vi "Function_Yellow Spot.vi"(0 "Image Src In":T4, 5 "Data Cluster In":cluster{"Name":string, "Variant In":variant}, 7 "CoordSys In":T1 {"Measurement System"."Axis Reference" items=["Direct", "Indirect"]; "Measurement System"."Angle (deg)" format="%.2f"; "Measurement System"."Origin"."Y" format="%.2f"; "Measurement System"."Origin"."X" format="%.2f"; "Reference System"."Axis Reference" items=["Direct", "Indirect"]; "Reference System"."Angle (deg)" format="%.2f"; "Reference System"."Origin"."Y" format="%.2f"; "Reference System"."Origin"."X" format="%.2f"}, 9 "Center(Annulus)":cluster{"X":sgl, "Y":sgl} {"Y" format="%.2f"; "X" format="%.2f"}, 11 "Error in":errorcluster) -> (4 "Objects":T3(array[cluster]) {"Area" format="%.2f"; "Object Center"."Y" format="%.2f"; "Object Center"."X" format="%.2f"}, 6 "Result(Yellow)":cluster{"Name":string, "NG?":bool, "Score":dbl}, 10 "ROI Out":T2 {"Contours"."Type" items=["No Selection", "Point", "Line", "Rectangle", "Oval", "Polygon", "Free", "Annulus", "Unused2", "Unused3", "Broken Line", "Free Hand Line", "Rotated Rectangle"]}, 14 "Time":u32, 15 "Error out":errorcluster)   [LabVIEW 2013]
uses:
  <vilib>/vision/Image Controls.llb/IMAQ Image.ctl
  Control/Control_Yellow Spot.ctl
  <vilib>/vision/NI_Vision_Development_Module.lvlib
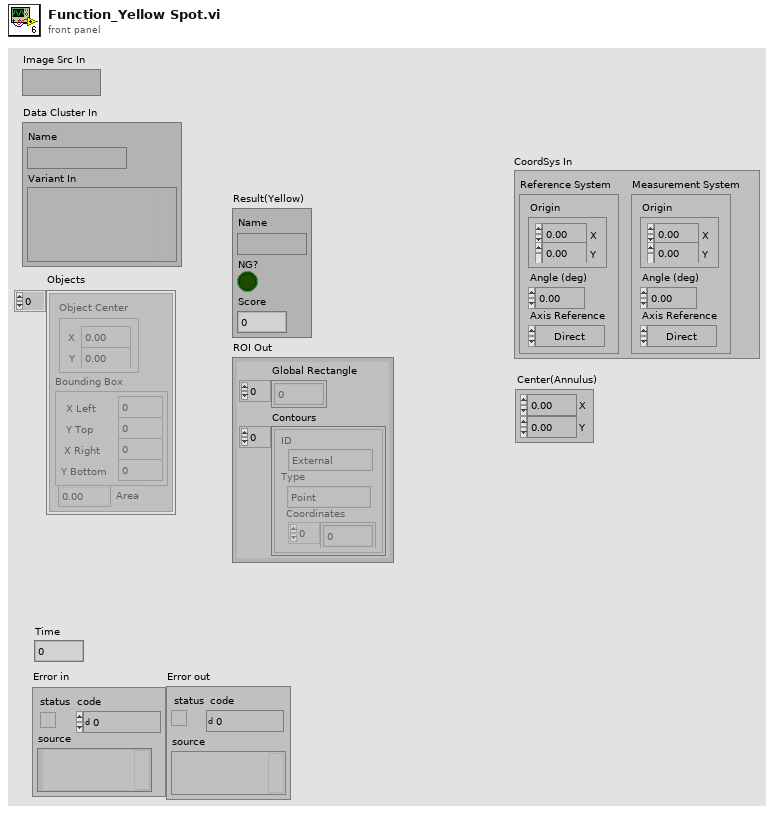
[diagram p1: front panel]
types:
  T1 = typedef "IMAQ Coordinate System" = cluster{"Reference System":cluster{"Origin":cluster{"X":sgl, "Y":sgl}, "Angle (deg)":sgl, "Axis Reference":u32}, "Measurement System":cluster{"Origin":cluster{"X":sgl, "Y":sgl}, "Angle (deg)":sgl, "Axis Reference":u32}}
  T2 = cluster{"Global Rectangle":i32[], "Contours":cluster{"ID":enum32{"External", "Internal"}, "Type":u32, "Coordinates":i32[]}[]}
  T3 = cluster{"Object Center":cluster{"X":dbl, "Y":dbl}, "Bounding Box":cluster{"X Left":dbl, "Y Top":dbl, "X Right":dbl, "Y Bottom":dbl}, "Area":dbl}[]
  T4 = typedef "IMAQ Image.ctl" = refnum<image>
  T5 = typedef "Control_Yellow Spot.ctl" = cluster{"Name":string, "ROI":cluster{"Global Rectangle":i32[], "Contours":cluster{"ID":enum32{"External", "Internal"}, "Type":u32, "Coordinates":i32[]}[]}, "Magnification(独闯)":i32, "»Ö­È(¶À´³)":i16, "Settings(独闯)":cluster{"Objects":enum16{"Bright Objects", "Dark Objects"}, "Threshold":i32, "Min Object Size":bool, "Min Size":i32, "Max Object Size":bool, "Max Size":i32}}
  T6 = cluster{"Objects":enum16{"Bright Objects", "Dark Objects"}, "Threshold":i32, "Min Object Size":bool, "Min Size":i32, "Max Object Size":bool, "Max Size":i32}
  T7 = cluster{"ID":enum32{"External", "Internal"}, "Type":u32, "Coordinates":i32[]}[]
  T8 = cluster{"ID":enum32{"External", "Internal"}, "Type":u32, "Coordinates":i32[]}
  T9 = cluster{"Origin":cluster{"X":sgl, "Y":sgl}, "Angle (deg)":sgl, "Axis Reference":u32}
  T10 = typedef "ROI Descriptor" = cluster{"Global Rectangle":i32[], "Contours":cluster{"ID":enum32{"External", "Internal"}, "Type":u32, "Coordinates":i32[]}[]}
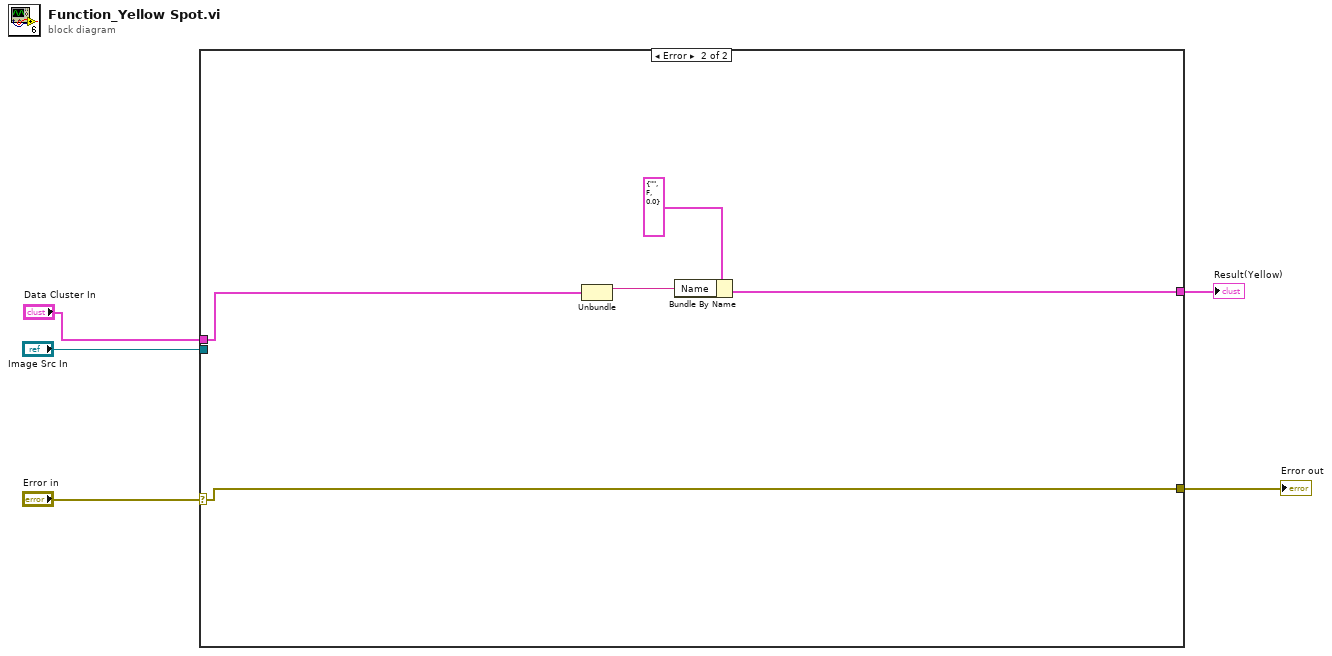
[diagram p0: block diagram]
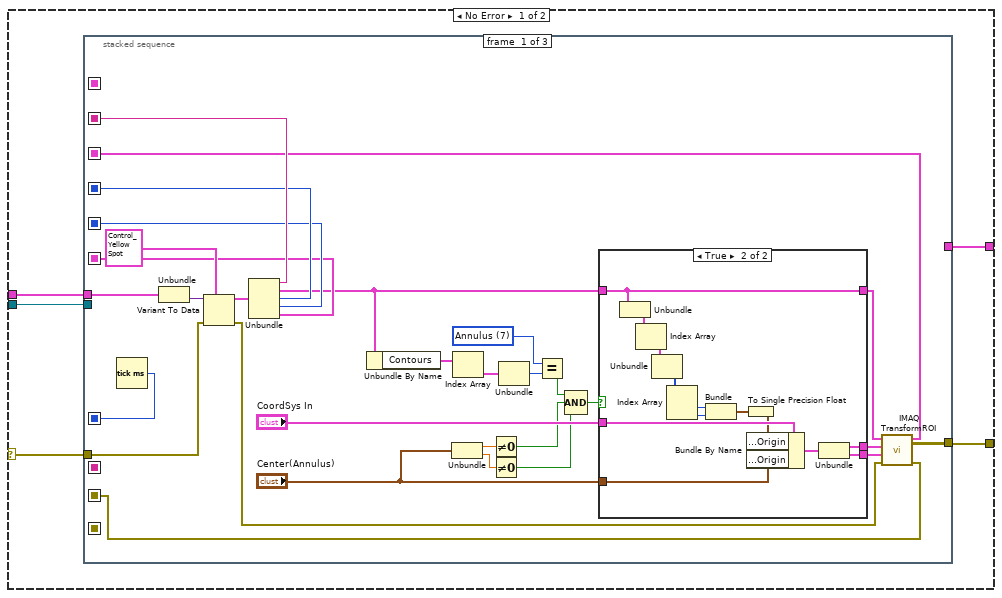
[diagram p2: hidden frame]
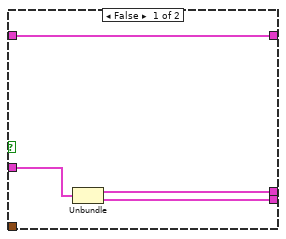
[diagram p3: hidden frame]
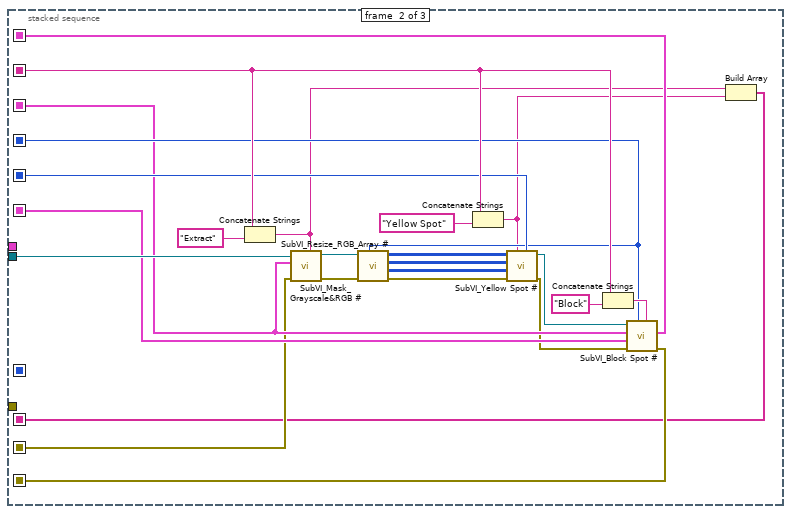
[diagram p4: hidden frame]
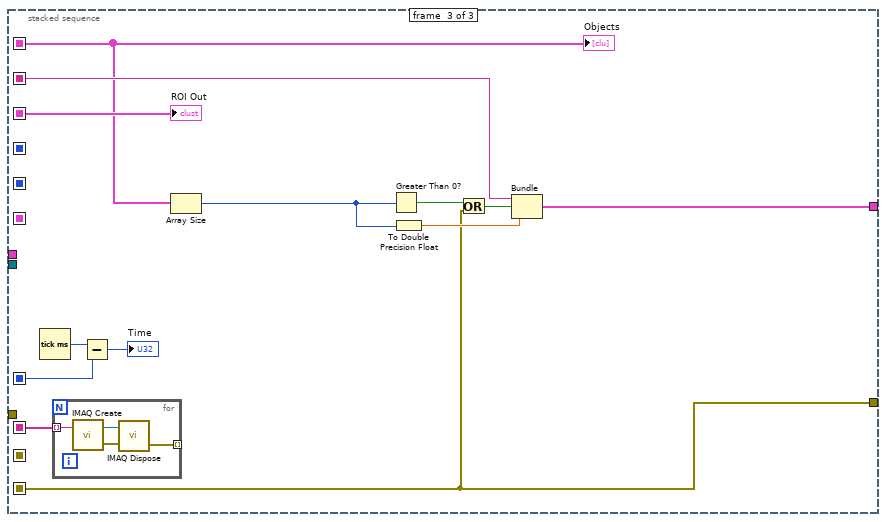
[diagram p5: hidden frame]
diagram:
  n1 = case shown="Error" "Error in" {
    selector: "Error in" -> [w8 w102]
    tunnel: [w10 w102] -> w5
    tunnel: "Image Src In" -> [w9 _]
    tunnel: [w7 w98] -> w2
    tunnel: "Data Cluster In" -> [w6 w99]
    frame No Error {
      n2 = stacked-sequence {
        seq-local: [w36 _ _] -> [_ w68 w90]
        seq-local: [w23 _ _] -> [_ w64 w91]
        seq-local: [w35 _ _] -> [_ w66 _]
        seq-local: [w34 _ _] -> [_ w67 _]
        seq-local: [w33 _ _] -> [_ w65 _]
        seq-local: [_ w62 _] -> [_ _ w86]
        seq-local: [_ w61 _] -> [_ _ w89]
        seq-local: [w32 _ _] -> [_ _ w84]
        seq-local: [w12 _ _] -> [_ w60 _]
        seq-local: [_ w57 _] -> [_ _ w82]
        tunnel: w8 -> [w14 _ _]
        tunnel: [_ _ w86] -> w10
        tunnel: w9 -> [_ w73 _]
        tunnel: [_ _ w81] -> w7
        tunnel: w6 -> [w11 _ _]
        frame #0 {
          w28 = u32 7 items=["No Selection", "Point", "Line", "Rectangle", "Oval", "Polygon", "Freehand Region", "Annulus", "Unused2", "Unused3", "Broken Line", "Freehand Line", "Rotated Rectangle"] ("Type")
          n3 = Tick Count (ms)() -> (millisecond timer value=w32:u32)
          n4 = Unbundle(w11) -> ("Variant In"=w38:variant)  [unwired: 1 out]
          n5 = Variant To Data(error in=w14, type=T5 {"Name"="", "ROI"={"Global Rectangle"=[], "Contours"=[]}, "Magnification(独闯)"=0, "»Ö­È(¶À´³)"=40, "Settings(独闯)"={"Objects"=enum."Bright Objects", "Threshold"=128, "Min Object Size"=FALSE, "Min Size"=3, "Max Object Size"=FALSE, "Max Size"=100}} ("独闯_Setting"), Variant=w38) -> (data=w37:T5, error out=w13:errorcluster)
          n6 = Unbundle(w37) -> ("Name"=w36:string, "ROI"=w24:T2, "Magnification(独闯)"=w35:i32, "»Ö­È(¶À´³)"=w34:i16, "Settings(独闯)"=w33:T6)
          n7 = Unbundle By Name(w24) -> ("Contours"=w26:T7)
          n8 = Unbundle("Center(Annulus)") -> ("X"=w20:sgl, "Y"=w19:sgl)
          n9 = Index Array(array=w26) -> (element=w27:T8)  [unwired: 1 in]
          n10 = Not Equal To 0?(x=w20) -> (x != 0?=w17:bool)
          n11 = Not Equal To 0?(x=w19) -> (x != 0?=w16:bool)
          n12 = Unbundle(w27) -> ("Type"=w29:u32)  [unwired: 2 out]
          n13 = Equal?(x=w28, y=w29) -> (x = y?=w18:bool)
          n14 = Compound Arithmetic op=AND(w18, w17, w16) -> (w15:bool)
          n15 = case shown="True" w15 {
            tunnel: "CoordSys In" -> [w43 w56]
            tunnel: [w42 w50] -> w30
            tunnel: [w41 w49] -> w31
            tunnel: "Center(Annulus)" -> [_ w53]
            tunnel: w24 -> [w40 w44]
            tunnel: [w40 w44] -> w22
            frame False {
              n16 = Unbundle(w43) -> ("Reference System"=w42:T9, "Measurement System"=w41:T9)
            }
            frame True {
              n17 = Unbundle(w44) -> ("Contours"=w48:T7)  [unwired: 1 out]
              n18 = Index Array(array=w48) -> (element=w47:T8)  [unwired: 1 in]
              n19 = Unbundle(w47) -> ("Coordinates"=w46:i32[])  [unwired: 2 out]
              n20 = Index Array(array=w46) -> (element #1=w55:i32, element #2=w54:i32)  [unwired: 2 in]
              n21 = Bundle(w55, w54) -> (w45:cluster{i32, i32})  [unwired: 1 in]
              n22 = To Single Precision Float(number=w45) -> (single precision float=w52:cluster{sgl, sgl})
              n23 = Bundle By Name(cluster=w56, "Reference System.Origin"=w52, "Measurement System.Origin"=w53) -> (w51:T1)
              n24 = Unbundle(w51) -> ("Reference System"=w50:T9, "Measurement System"=w49:T9)
            }
          }
          n25 = call "IMAQ TransformROI"("error in (no error)"=w13, "New Reference"=w31, "Base Reference"=w30, "ROI Descriptor"=w22) -> ("error out"=w12:errorcluster, "ROI Descriptor out"=w23:T10)  [unwired: 6 in]
        }
        frame #1 {
          n26 = Concatenate Strings(w68, "Extract" ("Image Register Name")) -> (w59:string)
          n27 = call "SubVI_Mask_Grayscale&RGB #.vi"("Image Register Name"=w59, "Error in"=w60, "ROI Descriptor"=w64, "Image Src In"=w73) -> ("Error out"=w76:errorcluster, "Image Dst Out"=w80:T4)  [unwired: 4 in, 2 out]
          n28 = call "SubVI_Resize_RGB_Array #.vi"("Magnification"=w66, "Error In"=w76, "Image In"=w80) -> ("Error Out"=w75:errorcluster, "B"=w79:u8[][], "G"=w78:u8[][], "R"=w74:u8[][])  [unwired: 5 in]
          n29 = Concatenate Strings(w68, "Yellow Spot" ("Image Register Name")) -> (w58:string)
          n30 = call "SubVI_Yellow Spot #.vi"("»Ö­È"=w67, "Image Register Name"=w58, "Error In"=w75, "B"=w79, "G"=w78, "R"=w74) -> ("Error Out"=w63:errorcluster, "Image Dst Out"=w77:T4)  [unwired: 4 in]
          n31 = Concatenate Strings(w68, "Block" ("Image Register Name")) -> (w70:string)
          n32 = call "SubVI_Block Spot #.vi"("Image Register Name"=w70, "Magnification"=w66, "Error in"=w63, "Settings"=w65, "ROI Descriptor"=w64, "Image Src In"=w77) -> ("Error out"=w62:errorcluster, "Objects"=w61:T3)  [unwired: 3 in, 1 out]
          n33 = Build Array(w59, w58) -> (w57:string[])
        }
        frame #2 {
          n34 = Tick Count (ms)() -> (millisecond timer value=w85:u32)
          n35 = for {
            tunnel: w82 -> [w97] mode=indexing
            tunnel: [w94] -> _ mode=indexing
            n36 = call "IMAQ Create"("Image Name"=w97) -> ("New Image"=w96:T4, "error out"=w95:errorcluster)  [unwired: 4 in]
            n37 = call "IMAQ Dispose"("Image"=w96, "error in (no error)"=w95) -> ("error out"=w94:errorcluster)  [unwired: 4 in]
          }
          n38 = Subtract(x=w85, y=w84) -> (x-y=→"Time":u32)
          n39 = Array Size(array=w89) -> (size(s)=w93:i32)
          n40 = Greater Than 0?(x=w93) -> (x > 0?=w87:bool)
          n41 = To Double Precision Float(number=w93) -> (double precision float=w92:dbl)
          n42 = Or(x=w87, y=w86) -> (x .or. y?=w88:bool)
          n43 = Bundle("Name"=w90, w88, w92) -> (w81:cluster{"Name":string, bool, dbl})  [unwired: 1 in]
          "Objects" <- w89
          "ROI Out" <- w91
        }
      }
    }
    frame Error {
      n44 = Unbundle(w99) -> ("Name"=w100:string)  [unwired: 1 out]
      n45 = Bundle By Name(cluster=cluster{"Name":string, bool, "Radius":dbl} {"Name"="", FALSE, "Radius"=0.0}, "Name"=w100) -> (w98:cluster{"Name":string, bool, "Radius":dbl})
    }
  }
  "Error out" <- w5
  "Result(Yellow)" <- w2
